vi "Actor Core.vi"(8 "error in":errorcluster, 11 "HIJ Vision App IMAQdx Display In":refnum<class "HIJ Vision Camera App w Timer.lvclass">) -> (0 "error out":errorcluster, 3 "Actor out":refnum<class "Actor.lvclass">)   [LabVIEW 2014, in "HIJ Vision Camera App w Timer.lvlib" / "HIJ Vision Camera App w Timer.lvclass"]
doc: "(<B>Filename</B>: Actor Framework.lvlib:Actor.lvclass:Actor Core.vi)\n\nReceives messages to the actor, reacts to them, and initiates any error handling that may shut the actor down.\n\nDescendant classes may override this VI to append parallel tasks for the actor to complete while it handles messages. Overrides use the Call Parent Method node."
uses:
  HIJ Vision Camera App w Timer.lvclass
  <vilib>/ActorFramework/Actor/Actor.lvclass
  Display Actors/HIJ IMAQdx Display/AF IMAQ Display/HIJ IMAQdx Display.lvclass
  Analyze/Analyze Classes/Analyze Diviation/Analyze BeamDeviation.lvclass
  Analyze/Results and Overlays/Results Beam Deviation/Analyze Results Beam Deviation.lvclass
  Analyze/Analyze Classes/Analyze Distanz/Analyze Distanz.lvclass
  Analyze/Results and Overlays/Results Distance/Analyze Results Distanz.lvclass
  Camera Actors/IMAQdx Actor/IMAQdx Actor/IMAQdx Actor.lvclass
  HIJ Vision Camera App w Timer Messages/Decrement ShotCounter Msg/Decrement ShotCounter Msg.lvclass
  Display Actors/HIJ Vision Display/HIJ Vision Display/HIJ Vision Display.lvclass/HIJ Vision Display.ctl
  HIJ Vision Camera App w Timer.lvclass/HIJ Vision Camera App w Timer.ctl
  Applications/HIJ Vision Application/HIJ Vision Application/HIJ Vision Application.lvclass/HIJ Vision Application.ctl
  Applications/HIJ Vision Camera App/HIJ Vision Camera App/HIJ Vision Camera App.lvclass/HIJ Vision Camera App.ctl
  Shared Code/Viewable Actor/ViewableActor/ViewableActor.lvclass/ViewableActor.ctl
  <vilib>/ActorFramework/Actor/Actor.lvclass/Actor.ctl
  <vilib>/ActorFramework/Message Enqueuer/Message Enqueuer.lvclass/Message Enqueuer.ctl
  Applications/HIJ Vision Camera App/HIJ Vision Camera App Messages/Menu Selection Msg/Menu Selection Msg.lvclass/Menu Selection Msg.ctl
  Display Actors/HIJ Vision Display/HIJ Vision Display/Write Save Report_.vi
  Applications/HIJ Vision Application/HIJ Vision Application/Write SubPnl for Display.vi
  Applications/HIJ Vision Camera App/HIJ Vision Camera App/Write Child Menu.vi
  Applications/HIJ Vision Application/HIJ Vision Application/Write HIJ Vision Display.vi
  Applications/HIJ Vision Application/HIJ Vision Application/Write Analyze Objs.vi
  Applications/HIJ Vision Camera App/HIJ Vision Camera App/Write Camera Actor.vi
  Shared Code/Viewable Actor/ViewableActor/Write UI VI Ref.vi
  <vilib>/ActorFramework/Message Enqueuer/Init from Existing Queue.vi
  <vilib>/ActorFramework/Message Enqueuer/Enqueue.vi
  <vilib>/ActorFramework/Message Priority Queue/Priority Enqueue.vi
  <vilib>/ActorFramework/Message Enqueuer/Message Enqueuer.lvclass
  Applications/HIJ Vision Camera App/HIJ Vision Camera App Messages/Menu Selection Msg/Menu Selection Msg.lvclass
  <vilib>/ActorFramework/Stop Msg/Stop Msg.lvclass
  Applications/HIJ Vision Camera App/HIJ Vision Camera App/HIJ Vision Camera App.lvclass
panel:
  out "next in":dbl
  in  "Stop Button":bool
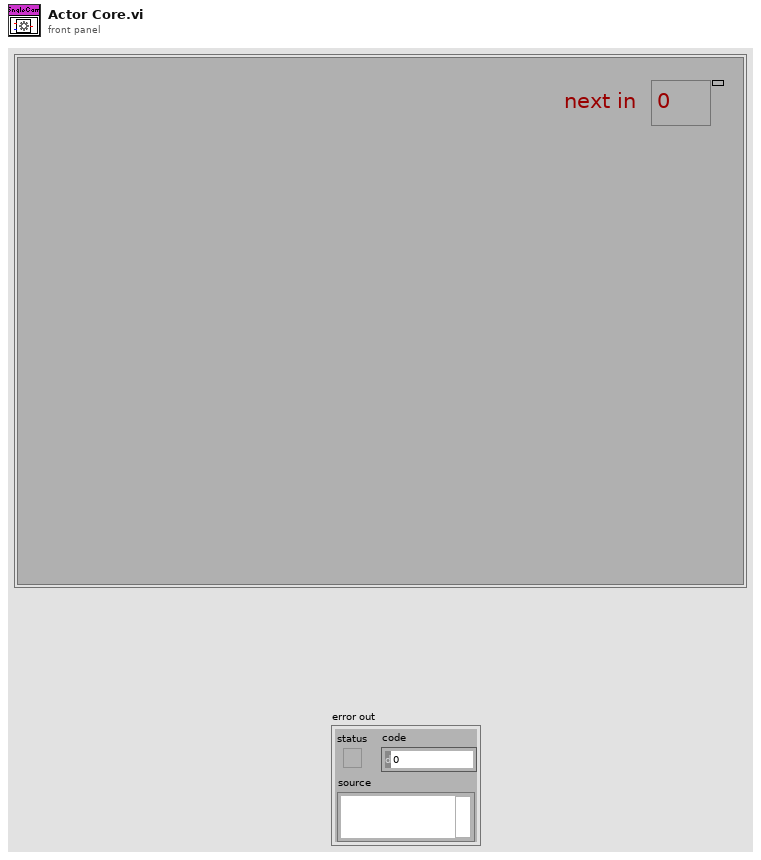
[diagram p1: front panel]
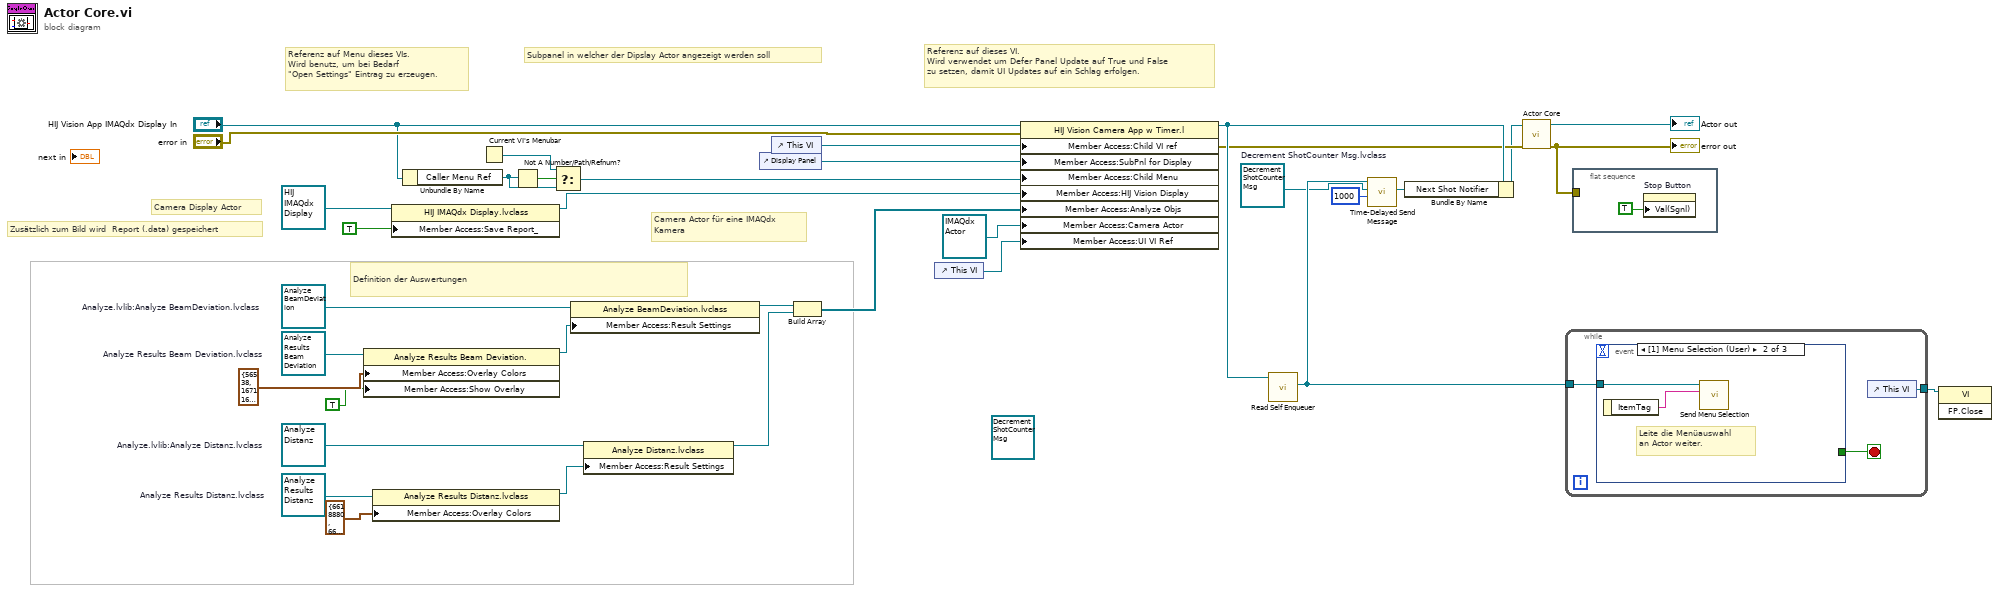
[diagram p0: block diagram]
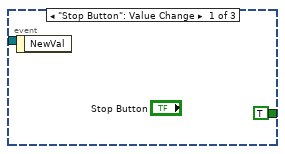
[diagram p2: hidden frame]
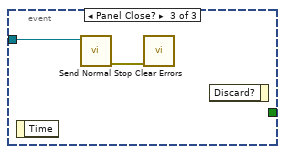
[diagram p3: hidden frame]
diagram:
  (unwired) refnum<class "Decrement ShotCounter Msg.lvclass"> refnum ("HIJ Vision Camera App w Timer.lvlib:Decrement ShotCounter Msg.lvclass")
  w1 = refnum<class "Decrement ShotCounter Msg.lvclass"> refnum  # Decrement ShotCounter Msg.lvclass
  w27 = refnum<class "Analyze Results Distanz.lvclass"> refnum  # Analyze Results Distanz.lvclass
  w28 = refnum<class "Analyze Distanz.lvclass"> refnum  # Analyze.lvlib:Analyze Distanz.lvclass
  w30 = refnum<class "Analyze Results Beam Deviation.lvclass"> refnum  # Analyze Results Beam Deviation.lvclass
  w31 = refnum<class "Analyze BeamDeviation.lvclass"> refnum  # Analyze.lvlib:Analyze BeamDeviation.lvclass
  # "Camera Actor für eine IMAQdx\nKamera"
  # "Referenz auf Menu dieses VIs.\nWird benutz, um bei Bedarf \n\"Open Settings\" Eintrag zu erzeugen."
  # "Referenz auf dieses VI.\nWird verwendet um Defer Panel Update auf True und False\nzu setzen, damit UI Updates auf ein Schlag erfolgen."
  # "Definition der Auswertungen"
  # "Camera Display Actor"
  # "Zusätzlich zum Bild wird  Report (.data) gespeichert"
  # "Subpanel in welcher der Dipslay Actor angezeigt werden soll"
  n1 = property class="Analyze Results Beam Deviation."(reference=w30, "Member Access:Overlay Colors"=cluster{"Border":u32, "Text":u32} {"Border"=56538, "Text"=16711680} ("Colors"), "Member Access:Show Overlay"=TRUE ("Show Overlay")) -> (reference out=w16:refnum<class "Analyze Results Beam Deviation.lvclass">)  [unwired: 1 in, 1 out]
  n2 = property class="Analyze Results Distanz.lvclass"(reference=w27, "Member Access:Overlay Colors"=cluster{"Border":u32, "Text":u32} {"Border"=6618880, "Text"=6618880} ("Colors")) -> (reference out=w15:refnum<class "Analyze Results Distanz.lvclass">)  [unwired: 1 in, 1 out]
  n3 = property class="HIJ IMAQdx Display.lvclass"(reference=refnum<class "HIJ IMAQdx Display.lvclass"> refnum ("IMAQ Display.lvlib:IMAQ Display.lvclass"), "Member Access:Save Report_"=TRUE ("Save Report_")) -> (reference out=w18:refnum<class "HIJ IMAQdx Display.lvclass">)  [unwired: 1 in, 1 out]
  n4 = Unbundle By Name("HIJ Vision App IMAQdx Display In") -> ("Caller Menu Ref"=w8:refnum<k9>)
  n5 = Current VI's Menubar() -> (w9:refnum<k9>)
  n6 = Not A Number/Path/Refnum?(number/path/refnum=w8) -> (NaN/Path/Refnum?=w11:bool)
  n7 = Select(t=w9, s=w11, f=w8) -> (s? t:f=w10:refnum<k9>)
  n8 = property class="Analyze BeamDeviation.lvclass"(reference=w31, "Member Access:Result Settings"=w16) -> (reference out=w17:refnum<class "Analyze BeamDeviation.lvclass">)  [unwired: 1 in, 1 out]
  n9 = property class="Analyze Distanz.lvclass"(reference=w28, "Member Access:Result Settings"=w15) -> (reference out=w14:refnum<class "Analyze Distanz.lvclass">)  [unwired: 1 in, 1 out]
  n10 = control-ref of="Display Panel"() -> (w20:refnum<vi>)
  n11 = control-ref of="This VI"() -> (w24:refnum<vi>)
  n12 = Build Array(w17, w14) -> (w21:refnum<class "Analyze BaseClass.lvclass">[])
  n13 = control-ref of="This VI"() -> (w13:refnum<vi>)
  n14 = property class="HIJ Vision Camera App w Timer.l"(reference="HIJ Vision App IMAQdx Display In", error in="error in", "Member Access:Child VI ref"=w24, "Member Access:SubPnl for Display"=w20, "Member Access:Child Menu"=w10, "Member Access:HIJ Vision Display"=w18, "Member Access:Analyze Objs"=w21, "Member Access:Camera Actor"=refnum<class "IMAQdx Actor.lvclass"> refnum ("IMAQdx Actor.lvlib:IMAQdx Actor.lvclass"), "Member Access:UI VI Ref"=w13) -> (reference out=w25:refnum<class "HIJ Vision Camera App w Timer.lvclass">, error out=w22:errorcluster)
  n15 = call <vilib>:"Read Self Enqueuer.vi"("Actor"=w25) -> ("Self Enqueuer"=w2:refnum<class "Message Enqueuer.lvclass">)  [unwired: 10 in]
  n16 = call <vilib>:"Time-Delayed Send Message.vi"("Milliseconds To Wait"=1000, "Message"=w1, "Message Enqueuer"=w2) -> ("Delivery Notifier"=w3:refnum<notifier>)  [unwired: 7 in, 1 out]
  n17 = Bundle By Name(cluster=w25, "Next Shot Notifier"=w3) -> (w4:refnum<class "HIJ Vision Camera App w Timer.lvclass">)
  n18 = call-parent "Actor Core.vi"("error in"=w22, "HIJ Vision Camera App In"=w4) -> ("error out"=w33:errorcluster, "Actor out"=→"Actor out":refnum<class "Actor.lvclass">)  [unwired: 8 in]
  "error out" <- w33
  n19 = while {
    tunnel: w2 -> [w37]
    tunnel: [w36] -> w6
    stop <- w38 stop-if-true
    n20 = event shown="[1] Menu Selection (User)" {
      selector: _ -> [_ _ _]
      dyn-events: _ -> [_ _ _]
      timeout: _ -> [_ _ _]
      tunnel: [TRUE _ _] -> w38
      tunnel: w37 -> [_ w40 w43]
      event "Stop Button": Value Change {
        n21 = event-data() -> ()  [unwired: 1 in, 1 out]
      }
      event Menu Selection (User) {
        # "Leite die Menüauswahl \nan Actor weiter."
        n22 = event-data() -> ("ItemTag"=w41:string)  [unwired: 1 in]
        n23 = call "Send Menu Selection.vi"("MenuTag"=w41, "Message Enqueuer"=w40) -> ()  [unwired: 8 in, 2 out]
      }
      event Panel Close? {
        n24 = event-data() -> ()  [unwired: 1 in, 1 out]
        n25 = call <vilib>:"Send Normal Stop.vi"("Message Enqueuer"=w43) -> ("error out"=w42:errorcluster)  [unwired: 10 in]
        n26 = call <vilib>:"Clear Errors.vi"("error in (no error)"=w42) -> ()  [unwired: 5 in, 2 out]
        n27 = event-data() -> ()  [unwired: 2 in, 1 out]
      }
    }
    n28 = control-ref of="This VI"() -> (w36:refnum<vi>)
  }
  n29 = flat-sequence {
    tunnel: w33 -> [_]
    frame #0 {
      n30 = property on="Stop Button" class="Bool (strict)"("Val(Sgnl)"=TRUE) -> ()  [unwired: 2 in, 2 out]
    }
  }
  n31 = invoke class="VI" method="FP.Close"(reference=w6) -> ()  [unwired: 2 in, 3 out]
